vi "TellComponent.vi"(9 "ActorAlias":string, 10 "Message":T1 {"MessageMetadata"."AbsoluteTime" format="%<%x %.3X>T"}, 11 "Actor":refnum<class "Actor.lvclass">) -> (3 "Actor":refnum<class "Actor.lvclass">)   [LabVIEW 2020, in "_Template.lvlib" / "MessageTemplate.lvlib" / "{{Name}}.lvlib"]
uses:
  {{Name}}.lvlib
  jettl/jettl/Actor/Actor.lvclass
  ConcreteMessage/ConcreteMessage.lvclass
  C:/jettl-harness/repos/jettl/src/jettl/jettl/Message/Message.lvclass
  jettl/jettl/Message/Message.lvclass
  jettl/jettl/jettl.lvlib
  jettl/jettl/Lifetime.ctl
  jettl/jettl/MessageMetadata.ctl
  Message.ctl
  jettl/jettl/TellOrigin.ctl
panel:
  # "This front panel should not be manipulated."
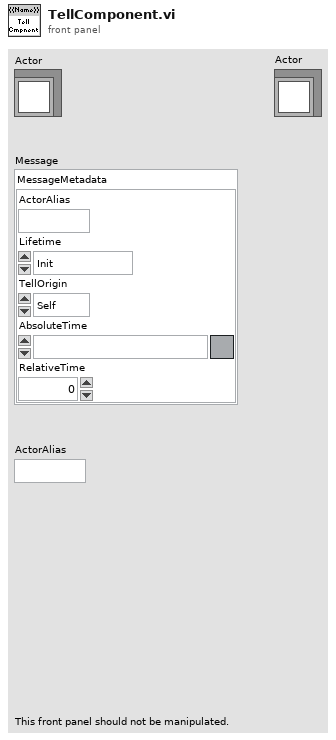
[diagram p1: front panel]
types:
  T1 = typedef "_Template.lvlib/MessageTemplate.lvlib/{{Name}}.lvlib/Message.ctl" = cluster{"MessageMetadata":T2}
  T2 = typedef "jettl.lvlib/MessageMetadata.ctl" = cluster{"ActorAlias":string, "Lifetime":T3, "TellOrigin":T4, "AbsoluteTime":timestamp, "RelativeTime":dbl}
  T3 = typedef "jettl.lvlib/Lifetime.ctl" = enum16{"Init", "Spawn", "Setup", "TeardownBeforeRunning", "Running", "StopCalled", "StoppingWithComponents", "StoppingNoComponents", "TeardownAfterRunning", "Stopped"}
  T4 = typedef "jettl.lvlib/TellOrigin.ctl" = enum16{"Self", "Mediator", "Component"}
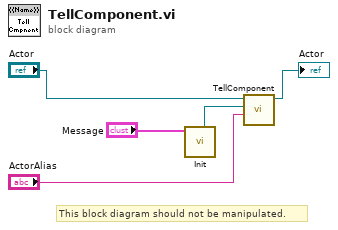
[diagram p0: block diagram]
diagram:
  # "This block diagram should not be manipulated."
  n1 = call "Init.vi"("Message"="Message") -> ("ConcreteMessage"=w3:refnum<class "ConcreteMessage.lvclass">)  [unwired: 10 in]
  n2 = call "TellComponent.vi"("ActorAlias"="ActorAlias", "Message"=w3, "Actor"="Actor") -> ("Actor"=→"Actor":refnum<class "Actor.lvclass">)  [unwired: 8 in]
